vi "SmartMotor_MotionStatus v4.vi"(0 "VISA In":refnum<visa-resource-name>, 1 "MotorSpecifier(M1)":T1=enum."M1", 5 "flush":bool, 7 "AuxStatusWordSelection(1)":i32(ring) items=["1", "2", "3", "4", "5", "6", "7", "8", "9", "10", "11", "12", "13", "14", "15", "16", "17"], 9 "Bypass(F)":bool, 11 "error in":errorcluster, 12 "Sem Timeout (5000)":i32=5000, 14 "ReadWait":u32=50) -> (3 "query cmds":string[](array[string]), 4 "VISA Out":refnum<visa-resource-name>, 6 "NumResults":dbl[](array[numeric]), 8 "SelectedAuxWord":dbl, 10 "StrRsp":string[](array[string]), 15 "error out":errorcluster)   [LabVIEW 2017]
doc: "Developed by Kevin Thompson\nkevin@thompsonengineering.net\n\nCopyright 2018-2020\nThompson Engineering, LLC"
uses:
  TD SerialBusMotorSpecifier_enum.ctl
  <vilib>/Instr/_visa.llb/VISA Flush IO Buffer Mask.ctl
panel:
  # "[0] RPA\n[1] REA\n[2] RVA\n[3] RW(0)\n[4] RW(..)"
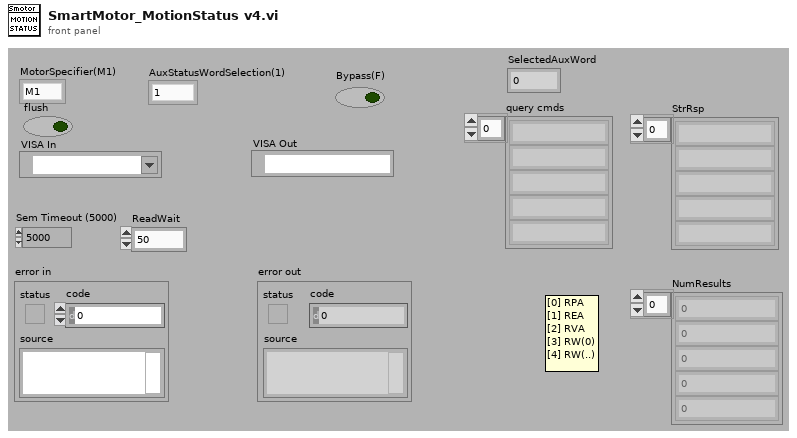
[diagram p1: front panel]
types:
  T1 = typedef "TD SerialBusMotorSpecifier_enum.ctl" = enum16{"None", "Global", "M1", "M2", "M3"}
  T2 = typedef "Semaphore RefNum" = refnum<k1>
  T3 = typedef "VISA Flush IO Buffer Mask.ctl" = u16
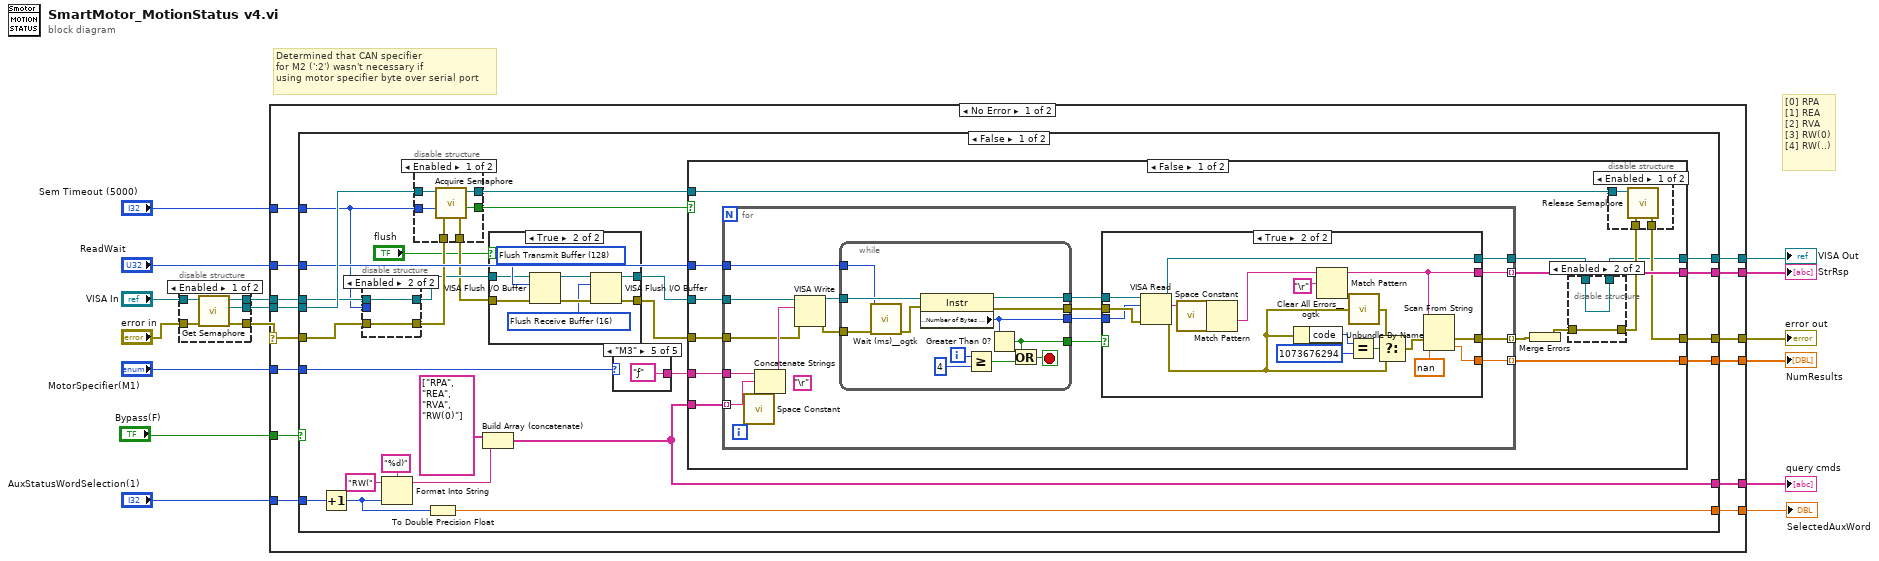
[diagram p0: block diagram]
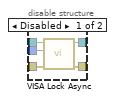
[diagram p4: hidden frame]
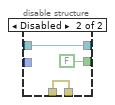
[diagram p5: hidden frame]
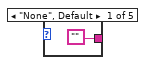
[diagram p6: hidden frame]
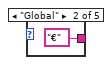
[diagram p7: hidden frame]
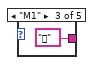
[diagram p8: hidden frame]
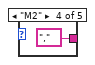
[diagram p9: hidden frame]
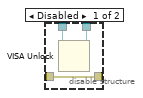
[diagram p10: hidden frame]
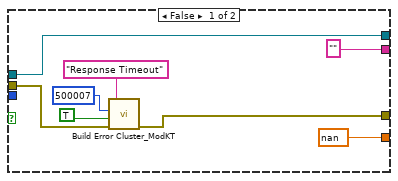
[diagram p12: hidden frame]
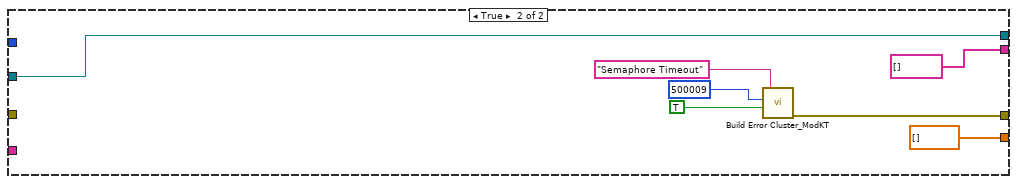
[diagram p13: hidden frame]
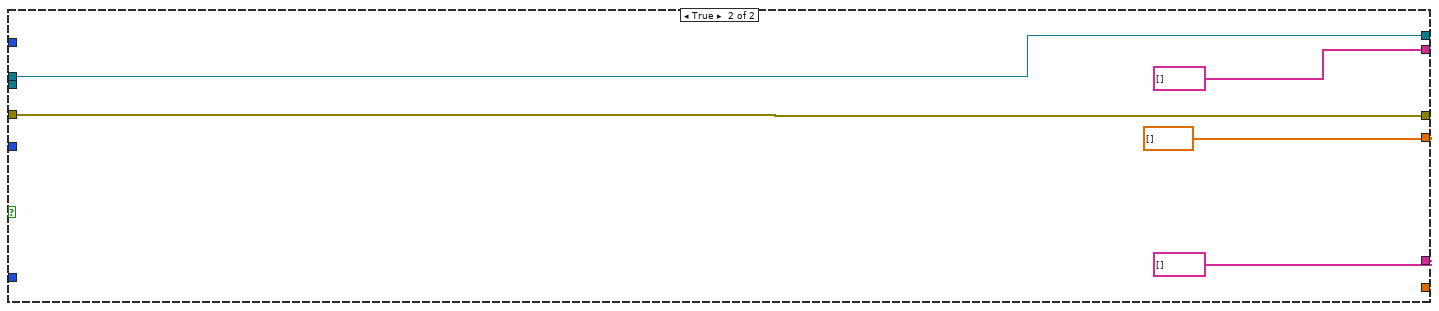
[diagram p14: hidden frame]
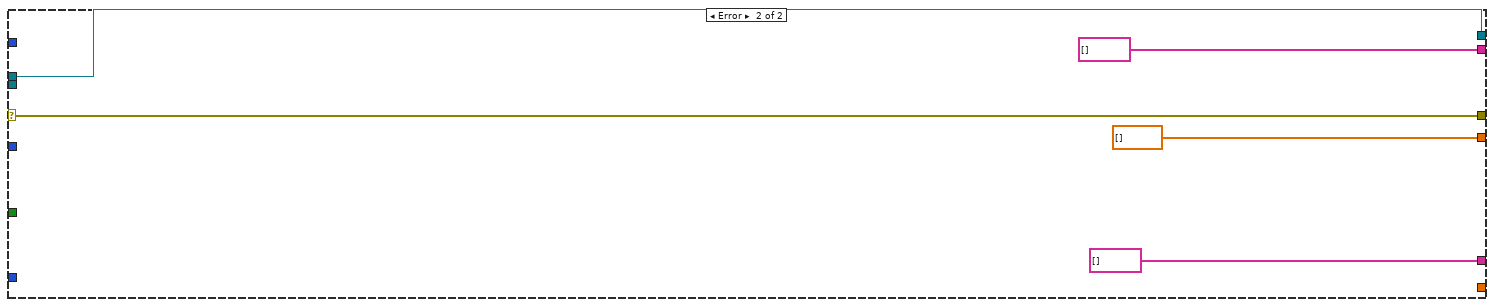
[diagram p15: hidden frame]
diagram:
  # "Determined that CAN specifier\nfor M2 (':2') wasn't necessary if\nusing motor specifier byte over serial port"
  # "[0] RPA\n[1] REA\n[2] RVA\n[3] RW(0)\n[4] RW(..)"
  n1 = disable-structure shown="Enabled" {
    disable-tunnel: [w21 w23] -> w9
    disable-tunnel: "VISA In" -> [w20 w23]
    disable-tunnel: [w19 w22] -> w7
    disable-tunnel: "error in" -> [w18 w22]
    disable-tunnel: [w17 _] -> w5
    frame Enabled {
      n2 = call "Get Semaphore.vi"("error in"=w18, "VISA In"=w20) -> ("error out"=w19:errorcluster, "semaphore out"=w17:T2, "VISA Out"=w21:refnum<visa-resource-name>)  [unwired: 3 in]
    }
    frame Disabled {
    }
  }
  n3 = case shown="No Error" w7 {
    selector: w7 -> [w32 w187]
    tunnel: w9 -> [w37 w190]
    tunnel: [w30 string[] []] -> w16
    tunnel: [w36 w187] -> w15
    tunnel: [w35 w190] -> w14
    tunnel: [w34 dbl[] []] -> w13
    tunnel: [w33 string[] []] -> w12
    tunnel: "AuxStatusWordSelection(1)" -> [w31 _]
    tunnel: "Bypass(F)" -> [w29 _]
    tunnel: w5 -> [w28 _]
    tunnel: "Sem Timeout (5000)" -> [w27 _]
    tunnel: "MotorSpecifier(M1)" -> [w26 _]
    tunnel: "ReadWait" -> [w25 _]
    tunnel: [w24 _] -> w1
    frame No Error {
      n4 = case shown="False" w29 {
        tunnel: w37 -> [w46 w185]
        tunnel: [w64 w184] -> w36
        tunnel: [w63 w185] -> w35
        tunnel: [w62 dbl[] []] -> w34
        tunnel: [w61 string[] []] -> w33
        tunnel: w32 -> [w45 w184]
        tunnel: w31 -> [w51 _]
        tunnel: [w49 string[] []] -> w30
        tunnel: w28 -> [w60 _]
        tunnel: w27 -> [w43 _]
        tunnel: w26 -> [w57 _]
        tunnel: w25 -> [w55 _]
        tunnel: [w47 _] -> w24
        frame False {
          n5 = Increment(x=w51) -> (x+1=w48:i32)
          n6 = disable-structure shown="Enabled" {
            disable-tunnel: w46 -> [w79 w80]
            disable-tunnel: [w78 w80] -> w42
            disable-tunnel: w45 -> [w77 w81]
            disable-tunnel: [w76 w81] -> w44
            disable-tunnel: w43 -> [w75 _]
            frame Disabled {
              n7 = call <vilib>:"VISA Lock Async.vi"("error in (no error)"=w77, "timeout (0)"=w75, "VISA resource name"=w79) -> ("error out"=w76:errorcluster, "VISA resource name out"=w78:refnum<visa-resource-name>)  [unwired: 6 in, 1 out]
            }
            frame Enabled {
            }
          }
          n8 = Format Into String(format string="%d)", initial string="RW(", w48) -> (resulting string=w50:string)  [unwired: 1 in, 1 out]
          n9 = disable-structure shown="Enabled" {
            disable-tunnel: w60 -> [w87 w89]
            disable-tunnel: [w86 FALSE ("timed out")] -> w59
            disable-tunnel: [w85 w89] -> w58
            disable-tunnel: w44 -> [w84 w90]
            disable-tunnel: [w83 w90] -> w40
            disable-tunnel: w43 -> [w82 _]
            frame Enabled {
              n10 = call <vilib>:"Acquire Semaphore.vi"("error in (no error)"=w84, "ms timeout (-1)"=w82, "semaphore"=w87) -> ("error out"=w83:errorcluster, "timed out"=w86:bool, "semaphore out"=w85:T2)  [unwired: 2 in]
            }
            frame Disabled {
            }
          }
          n11 = To Double Precision Float(number=w48) -> (double precision float=w47:dbl)
          n12 = Build Array (concatenate)(string[] ["RPA", "REA", "RVA", "RW(0)"], w50) -> (w49:string[])
          n13 = case shown="True" "flush" {
            tunnel: w42 -> [w66 w73]
            tunnel: [w65 w70] -> w39
            tunnel: [w66 w69] -> w41
            tunnel: w40 -> [w65 w67]
            frame False {
            }
            frame True {
              w68 = T3 16 items=["Flush Receive Buffer"=16, "Write Transmit Buffer to Device"=32, "Flush Receive Buffer (No I/O)"=64, "Flush Transmit Buffer"=128] ("Mask")
              w74 = T3 128 items=["Flush Receive Buffer"=16, "Write Transmit Buffer to Device"=32, "Flush Receive Buffer (No I/O)"=64, "Flush Transmit Buffer"=128] ("Mask")
              n14 = VISA Flush I/O Buffer(VISA resource name=w73, mask (16)=w74, error in (no error)=w67) -> (VISA resource name out=w71:refnum<visa-resource-name>, error out=w72:errorcluster)
              n15 = VISA Flush I/O Buffer(VISA resource name=w71, mask (16)=w68, error in (no error)=w72) -> (VISA resource name out=w69:refnum<visa-resource-name>, error out=w70:errorcluster)
            }
          }
          n16 = case shown="\"M3\"" w57 {
            tunnel: ["" "€" "" "‚" "ƒ"] -> w56
            frame "None", Default {
            }
            frame "Global" {
            }
            frame "M1" {
            }
            frame "M2" {
            }
            frame "M3" {
            }
          }
          n17 = case shown="False" w59 {
            tunnel: w41 -> [w109 w178]
            tunnel: w49 -> [w108 _]
            tunnel: [w104 w174] -> w64
            tunnel: [w98 w178] -> w63
            tunnel: [w106 dbl[] []] -> w62
            tunnel: [w107 string[] []] -> w61
            tunnel: w58 -> [w105 _]
            tunnel: w56 -> [w103 _]
            tunnel: w39 -> [w102 _]
            tunnel: w55 -> [w101 _]
            frame False {
              n18 = for {
                tunnel: w109 -> [w132]
                tunnel: w108 -> [w131] mode=indexing
                tunnel: [w134] -> w107 mode=indexing
                tunnel: [w135] -> w99
                tunnel: [w133] -> w97 mode=indexing
                tunnel: [w130] -> w106 mode=indexing
                tunnel: w102 -> [w120]
                tunnel: w103 -> [w129]
                tunnel: w101 -> [w122]
                (unwired) "\r"
                n19 = call <vilib>:"Space Constant.vi"() -> ("String"=w121:string)
                n20 = Concatenate Strings(w129, w131, w121) -> (w124:string)
                n21 = VISA Write(VISA resource name=w132, write buffer=w124, error in (no error)=w120) -> (VISA resource name out=w128:refnum<visa-resource-name>, error out=w123:errorcluster)  [unwired: 1 out]
                n22 = while {
                  tunnel: w128 -> [w147]
                  tunnel: w123 -> [w146]
                  tunnel: [w145] -> w127
                  tunnel: [w144] -> w119
                  tunnel: [w143] -> w126
                  tunnel: [w141] -> w125
                  tunnel: w122 -> [w136]
                  i -> [w140]
                  stop <- w137 stop-if-true
                  n23 = call <userlib>:"Wait (ms)__ogtk.vi"("error in (no error)"=w146, "milliseconds to wait"=w136) -> ("error out"=w142:errorcluster)  [unwired: 8 in, 1 out]
                  n24 = property class="Instr"(reference=w147, error in=w142) -> (reference out=w144:refnum<visa-resource-name>, error out=w145:errorcluster, "Serial Settings:Number of Bytes at Serial Port"=w143:u32)
                  n25 = Greater Or Equal?(x=w140, y=4) -> (x >= y?=w138:bool)
                  n26 = Greater Than 0?(x=w143) -> (x > 0?=w141:bool)
                  n27 = Or(x=w141, y=w138) -> (x .or. y?=w137:bool)
                }
                n28 = case shown="True" w125 {
                  tunnel: w127 -> [w154 w173]
                  tunnel: w119 -> [w152 w172]
                  tunnel: w126 -> [_ w171]
                  tunnel: [w153 w169] -> w133
                  tunnel: [w152 w158] -> w135
                  tunnel: [nan ("measVal") w168] -> w130
                  tunnel: ["" ("read buffer") w161] -> w134
                  frame False {
                    n29 = call <vilib>:"Build Error Cluster_ModKT .vi"("Prepend String (\"\")"="Response Timeout" ("Prepend String (\"\")"), "code"=500007, "error? (F)"=TRUE, "error in (no error)"=w154) -> ("error out"=w153:errorcluster)  [unwired: 3 in, 1 out]
                  }
                  frame True {
                    n30 = VISA Read(VISA resource name=w172, byte count=w171, error in (no error)=w173) -> (VISA resource name out=w158:refnum<visa-resource-name>, read buffer=w157:string, error out=w163:errorcluster)  [unwired: 1 out]
                    n31 = call <vilib>:"Space Constant.vi"() -> ("String"=w159:string)
                    n32 = Match Pattern(string=w157, regular expression=w159) -> (after substring=w156:string)  [unwired: 1 in, 3 out]
                    n33 = Unbundle By Name(w163) -> ("code"=w167:i32)
                    n34 = Match Pattern(string=w156, regular expression="\r") -> (before substring=w161:string)  [unwired: 1 in, 3 out]
                    n35 = Equal?(x=w167, y=1073676294 ("error code")) -> (x = y?=w165:bool)
                    n36 = call <userlib>:"Clear All Errors__ogtk.vi"("Error In"=w163) -> ("Error Out"=w164:errorcluster)  [unwired: 3 in]
                    n37 = Select(t=w164, s=w165, f=w163) -> (s? t:f=w162:errorcluster)
                    n38 = Scan From String(input string=w161, error in=w162, default 1=nan ("measVal")) -> (error out=w169:errorcluster, output 1=w168:dbl)  [unwired: 2 in, 2 out]
                  }
                }
              }
              n39 = Merge Errors(w97) -> (w96:errorcluster)
              n40 = disable-structure shown="Enabled" {
                disable-tunnel: w96 -> [w110 w113]
                disable-tunnel: [w110 w113] -> w100
                disable-tunnel: w99 -> [w112 w114]
                disable-tunnel: [w111 w114] -> w98
                frame Disabled {
                  n41 = VISA Unlock(11:w112) -> (3:w111:refnum<visa-resource-name>)  [unwired: 1 in, 1 out]
                }
                frame Enabled {
                }
              }
              n42 = disable-structure shown="Enabled" {
                disable-tunnel: w105 -> [w117 _]
                disable-tunnel: w100 -> [w116 w118]
                disable-tunnel: [w115 w118] -> w104
                frame Enabled {
                  n43 = call <vilib>:"Release Semaphore.vi"("error in (no error)"=w116, "semaphore"=w117) -> ("error out"=w115:errorcluster)  [unwired: 4 in, 1 out]
                }
                frame Disabled {
                }
              }
            }
            frame True {
              n44 = call <vilib>:"Build Error Cluster_ModKT .vi"("Prepend String (\"\")"="Semaphore Timeout" ("Prepend String (\"\")"), "code"=500009, "error? (F)"=TRUE) -> ("error out"=w174:errorcluster)  [unwired: 4 in, 1 out]
            }
          }
        }
        frame True {
        }
      }
    }
    frame Error {
    }
  }
  "VISA Out" <- w14
  "error out" <- w15
  "query cmds" <- w16
  "NumResults" <- w13
  "StrRsp" <- w12
  "SelectedAuxWord" <- w1
